vi "GamepadToRGB.vi"(8 "Z":dbl, 9 "X":dbl, 10 "Y":dbl format="%#_13g") -> ()   [LabVIEW 2016]
uses:
  <vilib>/Rock Robotics/WPI/ThirdParty/Sensors/CANifier/CTRE_CANifier_LEDChannel.ctl
panel:
  # "Inputs"
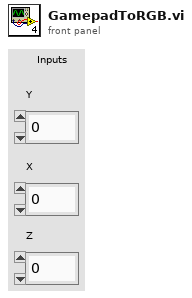
[diagram p1: front panel]
types:
  T1 = typedef "CTRE_CANifier_LEDChannel.ctl" = enum32{"LEDChannelA", "LEDChannelB", "LEDChannelC"}
  T2 = typedef "CTRE_CANifier_DeviceRef.ctl" = cluster{"DeviceStatus":errorcluster, "Device Number":u8, "Handle":u64, "UsageFrame":u32, "Library Path":path}
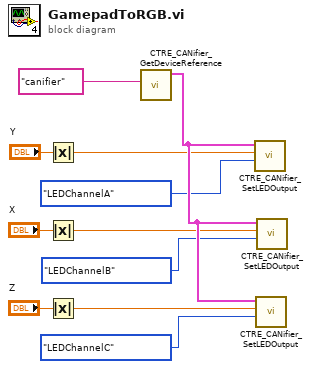
[diagram p0: block diagram]
diagram:
  n1 = Absolute Value(x="Y") -> (abs(x)=w6:dbl)
  n2 = Absolute Value(x="X") -> (abs(x)=w5:dbl)
  n3 = Absolute Value(x="Z") -> (abs(x)=w4:dbl)
  n4 = call <vilib>:"CTRE_CANifier_GetDeviceReference.vi"("refnum name"="canifier") -> ("CANifierDevRef"=w7:T2)  [unwired: 9 in, 1 out]
  n5 = call <vilib>:"CTRE_CANifier_SetLEDOutput.vi"("LEDChannel"=CTRE_CANifier_LEDChannel."LEDChannelA", "Percent Output"=w6, "CANifierDevRef"=w7) -> ()  [unwired: 7 in, 2 out]
  n6 = call <vilib>:"CTRE_CANifier_SetLEDOutput.vi"("LEDChannel"=CTRE_CANifier_LEDChannel."LEDChannelC", "Percent Output"=w4, "CANifierDevRef"=w7) -> ()  [unwired: 7 in, 2 out]
  n7 = call <vilib>:"CTRE_CANifier_SetLEDOutput.vi"("LEDChannel"=CTRE_CANifier_LEDChannel."LEDChannelB", "Percent Output"=w5, "CANifierDevRef"=w7) -> ()  [unwired: 7 in, 2 out]
